vi "Read Element JSON.vi"(8 "error in (no error)":errorcluster, 11 "ButtonControlEditorPanel in":refnum<class "ButtonControlEditorPanel.lvclass">) -> (0 "error out":errorcluster, 2 "JSON Props":T1, 3 "ButtonControlEditorPanel out":refnum<class "ButtonControlEditorPanel.lvclass">)   [LabVIEW 2020, in "VolatusGUIControls.lvlib" / "ButtonControlEditorPanel.lvclass"]
uses:
  ButtonControlEditorPanel.lvclass
  VolatusGUIControls.lvlib
  0389b728-1cf1-416b-bf2c-7d7cef5344ff.vi
  JSON Props.ctl
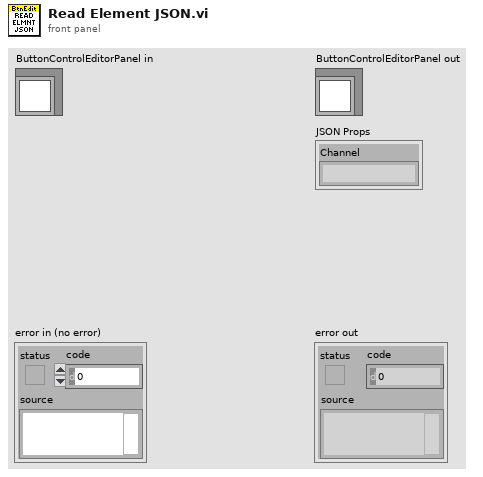
[diagram p1: front panel]
types:
  T1 = typedef "VolatusGUIControls.lvlib/ButtonControlEditorPanel.lvclass/JSON Props.ctl" = cluster{"Channel":string}
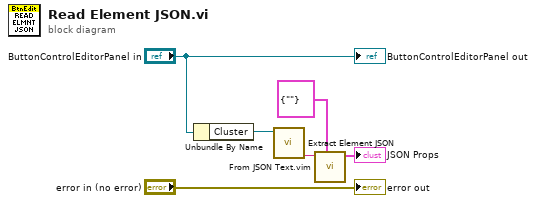
[diagram p0: block diagram]
diagram:
  n1 = Unbundle By Name("ButtonControlEditorPanel in") -> ("Cluster"=w4:refnum<vi>)
  n2 = call "Extract Element JSON.vi"("Ctl Refnum in"=w4) -> ("JSON"=w3:string)  [unwired: 7 in, 3 out]
  n3 = call "From JSON Text.vim"("Data Type and Default Value"=T1 {"Channel"=""}, "JSON"=w3) -> ("Data out"=→"JSON Props":T1)  [unwired: 8 in, 1 out]
  "error out" <- "error in (no error)"
  "ButtonControlEditorPanel out" <- "ButtonControlEditorPanel in"
